vi "Creat file for Seq path.vi"(11 "ini in":T4) -> (3 "Paths of Sequence":T1)   [LabVIEW 2018]
uses:
  type defs/Sequence paths.ctl
  type defs/Sequence Info.ctl
  type defs/Sequence Status.ctl
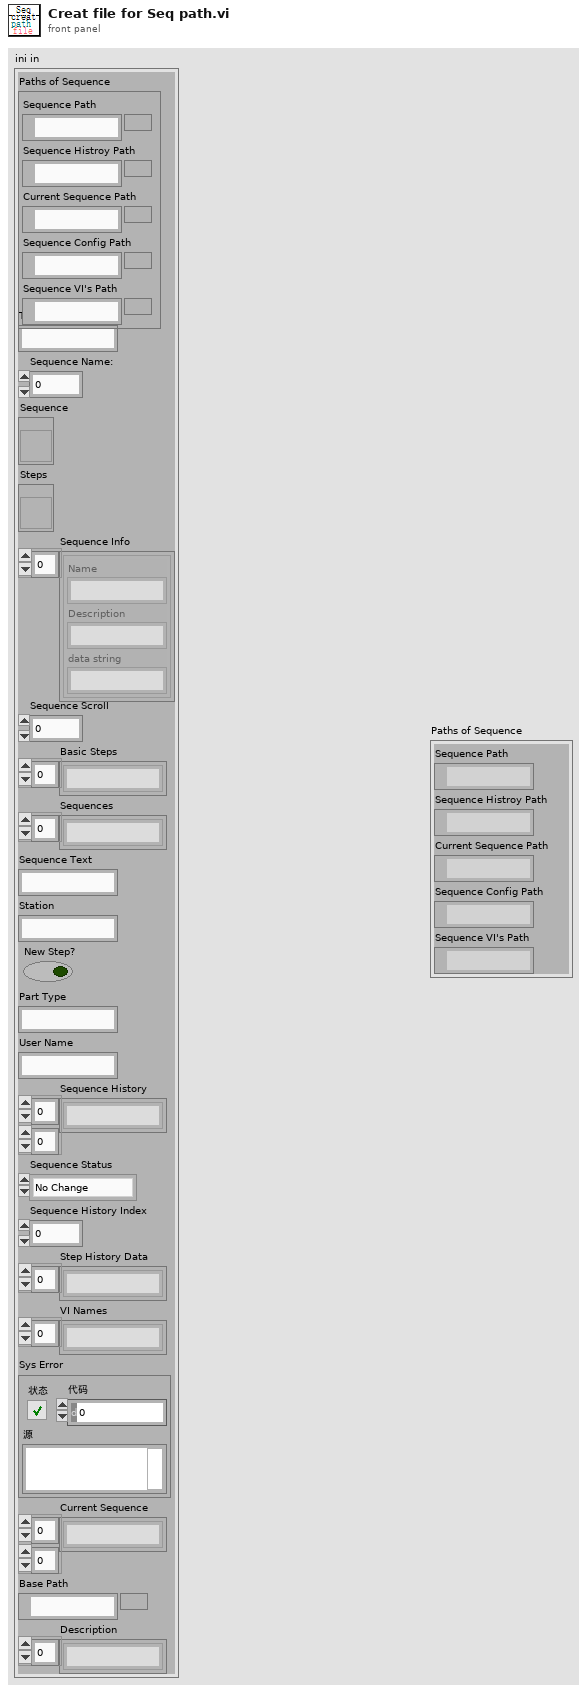
[diagram p1: front panel]
types:
  T1 = typedef "Sequence paths.ctl" = cluster{"Sequence Path":path, "Sequence Histroy Path":path, "Current Sequence Path":path, "Sequence Config Path":path, "Sequence VI's Path":path}
  T2 = typedef "Sequence Info.ctl" = cluster{"Name":string, "Description":string, "data string":string}
  T3 = typedef "Sequence Status.ctl" = enum16{"No Change", "Edited", "New Step", "Deleted", "Moved Up", "Moved Down", "Copied"}
  T4 = cluster{"Paths of Sequence":T1, "Type":string, "Sequence Name:":i32, "Sequence":refnum<vi>, "Steps":refnum<vi>, "Sequence Info":T2[], "Sequence Scroll":u32, "Basic Steps":string[], "Sequences":string[], "Sequence Text":string, "Station":string, "New Step?":bool, "Part Type":string, "User Name":string, "Sequence History":string[][], "Sequence Status":T3, "Sequence History Index":i32, "Step History Data":string[], "VI Names":string[], "Sys Error":errorcluster, "Current Sequence":string[][], "Base Path":path, "Description":string[]}
  T5 = enum16{"open", "replace", "create", "open or create", "replace or create", "replace or create with confirmation"}
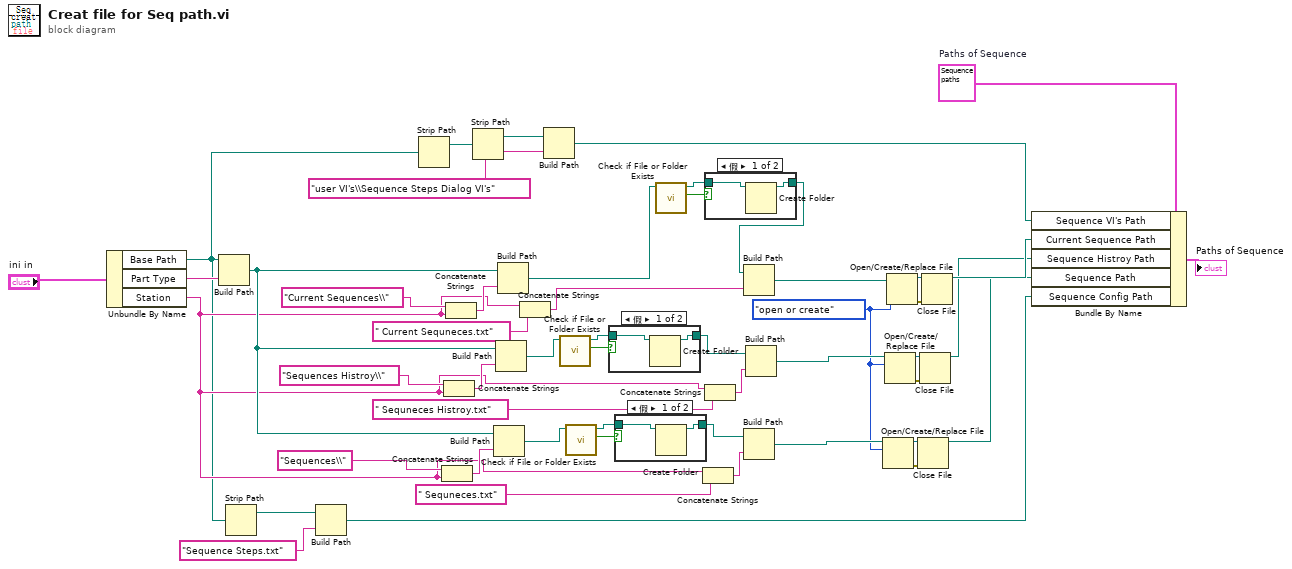
[diagram p0: block diagram]
diagram:
  w13 = T1 {"Sequence Path"=path "", "Sequence Histroy Path"=path "", "Current Sequence Path"=path "", "Sequence Config Path"=path "", "Sequence VI's Path"=path ""}  # Paths of Sequence
  w29 = T5."open or create" ("操作(0:open)")
  n1 = Unbundle By Name("ini in") -> ("Base Path"=w2:path, "Part Type"=w51:string, "Station"=w8:string)
  n2 = Build Path(base path=w2, name or relative path=w51) -> (appended path=w30:path)
  n3 = Strip Path(path=w2) -> (stripped path=w28:path)  [unwired: 1 out]
  n4 = Build Path(base path=w28, name or relative path="Sequence Steps.txt" ("名称或相对路径")) -> (appended path=w9:path)
  n5 = Strip Path(path=w2) -> (stripped path=w5:path)  [unwired: 1 out]
  n6 = Concatenate Strings("Sequences\\", w8) -> (w35:string)
  n7 = Concatenate Strings("Sequences Histroy\\", w8) -> (w42:string)
  n8 = Concatenate Strings("Current Sequences\\", w8) -> (w48:string)
  n9 = Strip Path(path=w5) -> (stripped path=w4:path)  [unwired: 1 out]
  n10 = Build Path(base path=w30, name or relative path=w35) -> (appended path=w15:path)
  n11 = Build Path(base path=w30, name or relative path=w42) -> (appended path=w19:path)
  n12 = Build Path(base path=w30, name or relative path=w48) -> (appended path=w23:path)
  n13 = Concatenate Strings(w8, " Current Sequneces.txt" ("字符串")) -> (w49:string)
  n14 = Build Path(base path=w4, name or relative path="user VI's\\Sequence Steps Dialog VI's" ("名称或相对路径")) -> (appended path=w1:path)
  n15 = call <vilib>:"Check if File or Folder Exists.vi"("path"=w19) -> ("file or folder exists?"=w21:bool, "dup path"=w20:path)  [unwired: 8 in, 1 out]
  n16 = call <vilib>:"Check if File or Folder Exists.vi"("path"=w15) -> ("file or folder exists?"=w17:bool, "dup path"=w16:path)  [unwired: 8 in, 1 out]
  n17 = case shown="假" w21 {
    tunnel: [w52 w54] -> w18
    tunnel: w20 -> [w53 w54]
    frame False {
      n18 = Create Folder(path (use dialog)=w53) -> (created path=w52:path)  [unwired: 2 in, 2 out]
    }
    frame True {
    }
  }
  n19 = case shown="假" w17 {
    tunnel: [w55 w57] -> w14
    tunnel: w16 -> [w56 w57]
    frame False {
      n20 = Create Folder(path (use dialog)=w56) -> (created path=w55:path)  [unwired: 2 in, 2 out]
    }
    frame True {
    }
  }
  n21 = call <vilib>:"Check if File or Folder Exists.vi"("path"=w23) -> ("file or folder exists?"=w26:bool, "dup path"=w25:path)  [unwired: 8 in, 1 out]
  n22 = Concatenate Strings(w8, " Sequneces.txt" ("字符串")) -> (w36:string)
  n23 = case shown="假" w26 {
    tunnel: [w58 w60] -> w22
    tunnel: w25 -> [w59 w60]
    frame False {
      n24 = Create Folder(path (use dialog)=w59) -> (created path=w58:path)  [unwired: 2 in, 2 out]
    }
    frame True {
    }
  }
  n25 = Concatenate Strings(w8, " Sequneces Histroy.txt" ("字符串")) -> (w43:string)
  n26 = Build Path(base path=w22, name or relative path=w49) -> (appended path=w24:path)
  n27 = Build Path(base path=w14, name or relative path=w36) -> (appended path=w33:path)
  n28 = Build Path(base path=w18, name or relative path=w43) -> (appended path=w40:path)
  n29 = Open/Create/Replace File(file path (use dialog)=w33, operation (0:open)=w29) -> (refnum out=w31:refnum<file>, error out=w32:errorcluster)  [unwired: 4 in, 1 out]
  n30 = Open/Create/Replace File(file path (use dialog)=w40, operation (0:open)=w29) -> (refnum out=w38:refnum<file>, error out=w39:errorcluster)  [unwired: 4 in, 1 out]
  n31 = Open/Create/Replace File(file path (use dialog)=w24, operation (0:open)=w29) -> (refnum out=w45:refnum<file>, error out=w46:errorcluster)  [unwired: 4 in, 1 out]
  n32 = Close File(refnum=w31, error in=w32) -> (path=w10:path)  [unwired: 1 out]
  n33 = Close File(refnum=w38, error in=w39) -> (path=w11:path)  [unwired: 1 out]
  n34 = Close File(refnum=w45, error in=w46) -> (path=w12:path)  [unwired: 1 out]
  n35 = Bundle By Name(cluster=w13, "Sequence VI's Path"=w1, "Current Sequence Path"=w12, "Sequence Histroy Path"=w11, "Sequence Path"=w10, "Sequence Config Path"=w9) -> (→"Paths of Sequence":T1)
